vi "Dispenser State.vi"(7 "Get/Set":enum16{"Get", "Set"}(ring), 8 "error in (no error)":errorcluster, 10 "New State":bool=TRUE, 11 "FlexWorktable in":refnum<class "FlexWorktable.lvclass">) -> (0 "error out":errorcluster, 2 "State":bool=TRUE, 3 "FlexWorktable out":refnum<class "FlexWorktable.lvclass">)   [LabVIEW 2017, in "FlexWorktable.lvclass"]
uses:
  FlexWorktable.lvclass
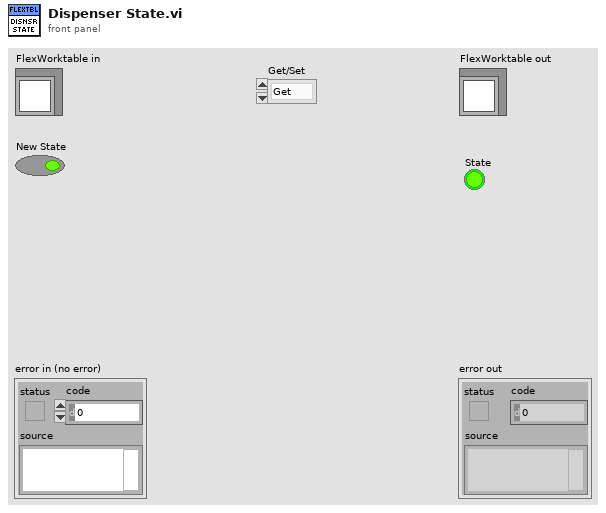
[diagram p1: front panel]
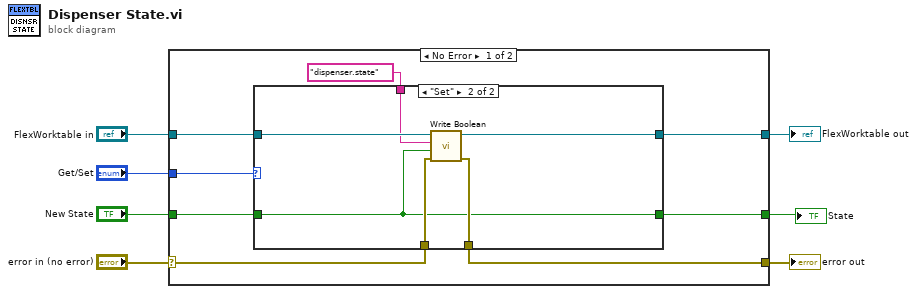
[diagram p0: block diagram]
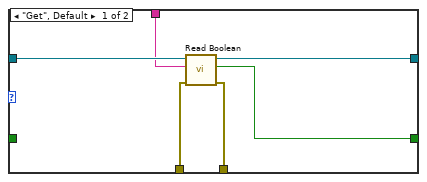
[diagram p2: hidden frame]
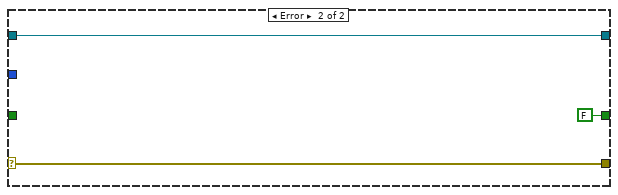
[diagram p3: hidden frame]
diagram:
  n1 = case shown="No Error" "error in (no error)" {
    selector: "error in (no error)" -> [w11 w30]
    tunnel: [w10 w30] -> w6
    tunnel: [w13 w29] -> w4
    tunnel: "FlexWorktable in" -> [w14 w29]
    tunnel: "New State" -> [w12 _]
    tunnel: "Get/Set" -> [w15 _]
    tunnel: [w9 FALSE ("New State")] -> w1
    frame No Error {
      n2 = case shown="\"Set\"" w15 {
        tunnel: w14 -> [w21 w27]
        tunnel: [w20 w26] -> w13
        tunnel: w12 -> [_ w23]
        tunnel: w11 -> [w17 w25]
        tunnel: [w16 w24] -> w10
        tunnel: [w18 w23] -> w9
        tunnel: "dispenser.state" ("Label") -> [w19 w22]
        frame "Get", Default {
          n3 = call-dynamic "Read Boolean.vi"("error in (no error)"=w17, "Label"=w19, "FlexWorktable in"=w21) -> ("error out"=w16:errorcluster, "Boolean"=w18:bool, "FlexWorktable out"=w20:refnum<class "FlexWorktable.lvclass">)  [unwired: 6 in]
        }
        frame "Set" {
          n4 = call-dynamic "Write Boolean.vi"("error in (no error)"=w25, "Boolean"=w23, "Label"=w22, "FlexWorktable in"=w27) -> ("error out"=w24:errorcluster, "FlexWorktable out"=w26:refnum<class "FlexWorktable.lvclass">)  [unwired: 6 in]
        }
      }
    }
    frame Error {
    }
  }
  "error out" <- w6
  "FlexWorktable out" <- w4
  "State" <- w1
